vi "Parse Variable Value Pairs.vi"(10 "Value":string[](array[string])=["{a:757.273473m;b:445.885196m}", "306", "18", "106", "206", "454.112"], 11 "Name":string[](array[string])=["cluster", "intfromini", "response", "response1", "response2", "cluster.a"]) -> (2 "Value":string[](array[string])=["cluster", "cluster.a", "cluster.b", "intfromini", "response", "response1", "response2", "cluster.a"], 3 "Name2":string[](array[string])=["cluster", "cluster.a", "cluster.b", "intfromini", "response", "response1", "response2", "cluster.a"])   [LabVIEW 2020]
uses:
  <userlib>/_NEVSTOP/Communicable State Machine(CSM)/Communicable State Machine.lvlib
  <userlib>/_NEVSTOP/Communicable State Machine(CSM)/_Shared/CSM Shared.lvlib
panel:
  out "Indexs 2":dbl[](array[numeric])=[5.0, 0.0, 2.0, 3.0, 4.0, 5.0, 1.0] format="%.2f"
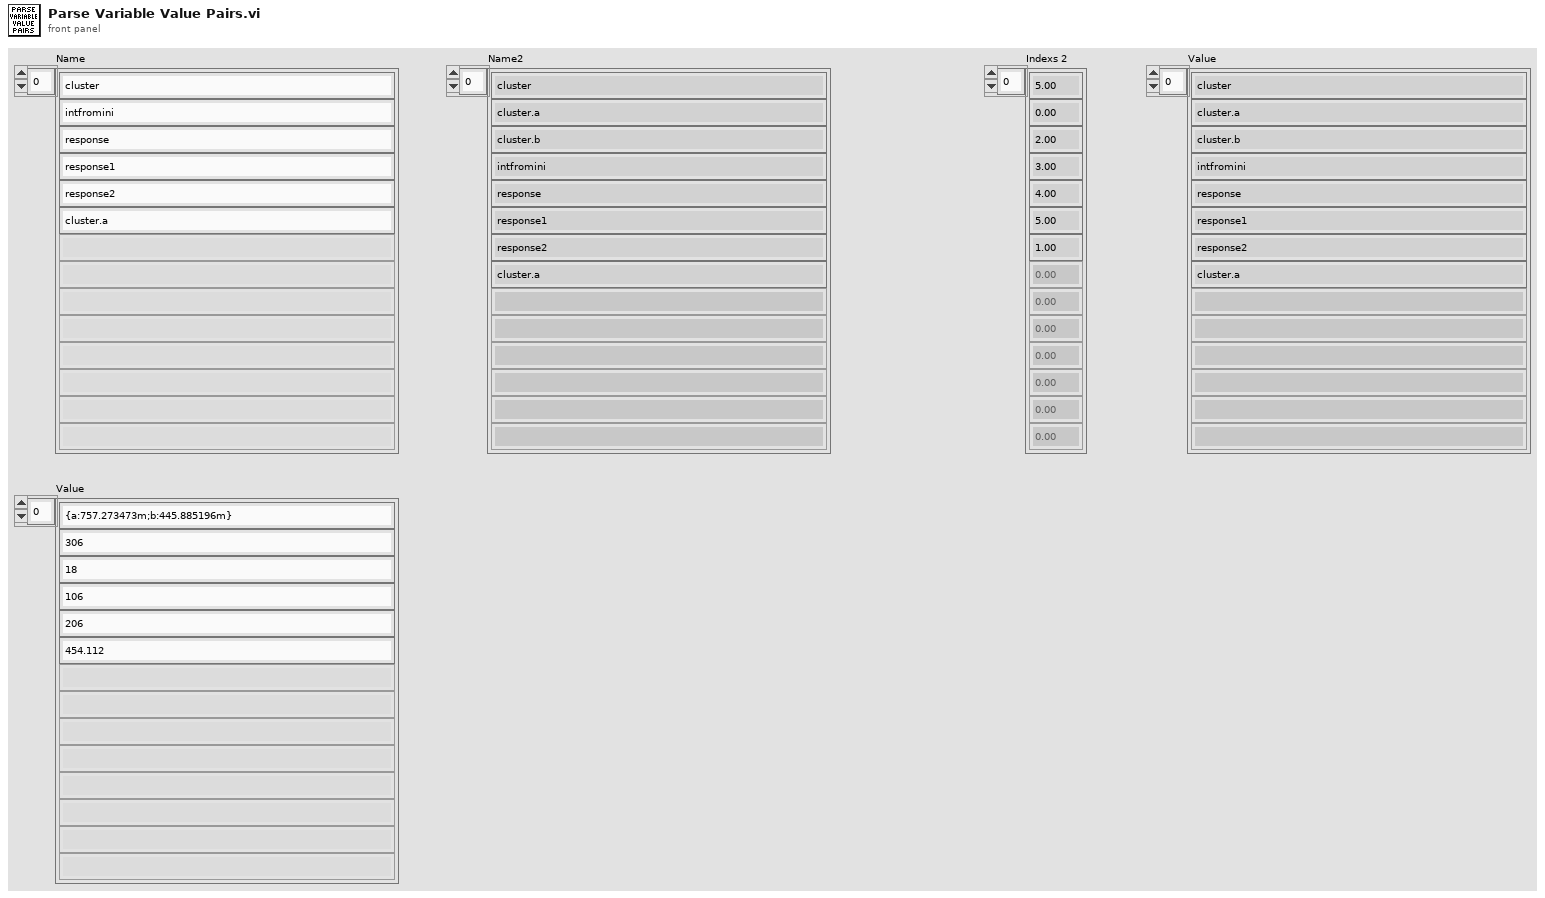
[diagram p1: front panel]
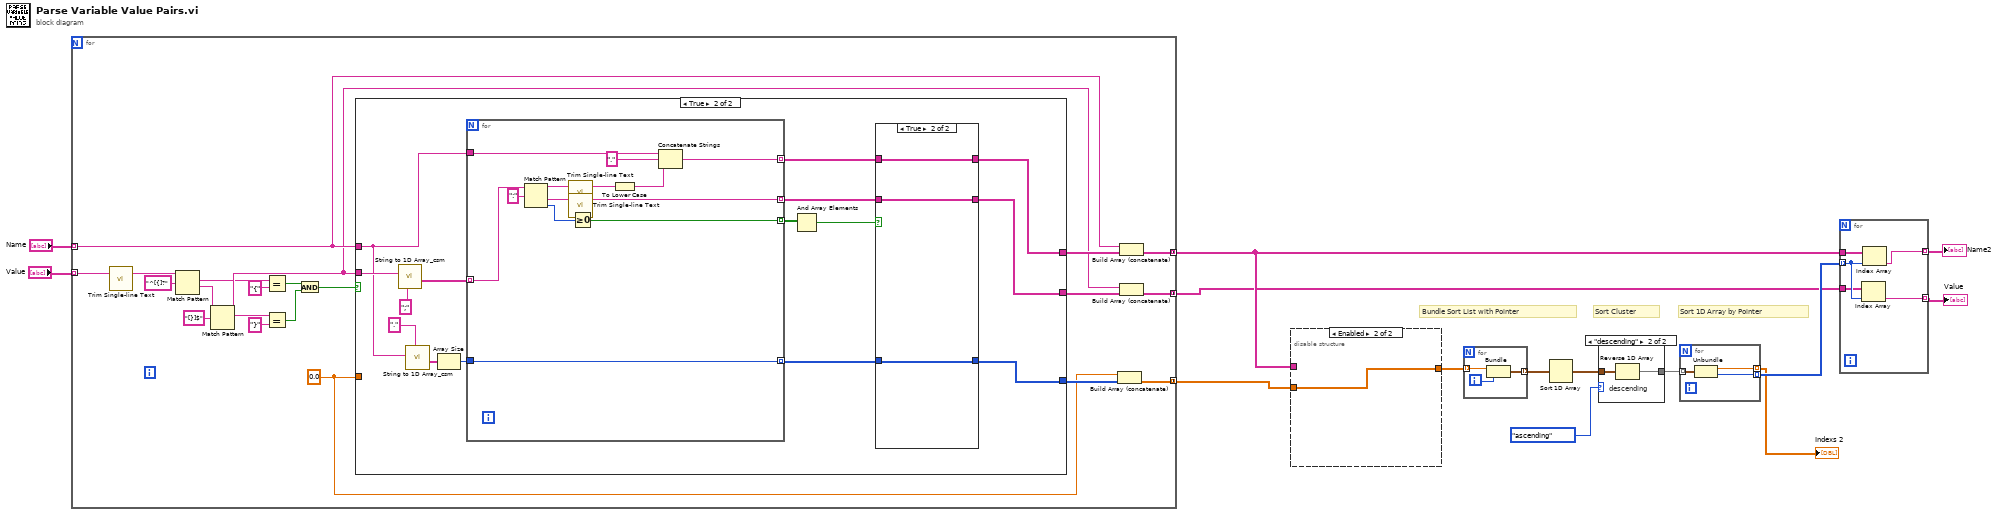
[diagram p0: block diagram]
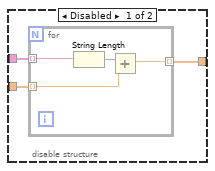
[diagram p2: hidden frame]
diagram:
  # "Sort 1D Array by Pointer"
  # "Sort Cluster"
  # "Bundle Sort List with Pointer"
  n1 = for {
    tunnel: "Value" -> [w35] mode=indexing
    tunnel: "Name" -> [w30] mode=indexing
    tunnel: [w32] -> w5 mode=concatenating
    tunnel: [w31] -> w2 mode=concatenating
    tunnel: [w23] -> w6 mode=concatenating
    w15 = 0.0 ("element")
    n2 = call <userlib>:"Trim Single-line Text.vi"("single-line text"=w35) -> ("trimed text"=w26:string)  [unwired: 2 in]
    n3 = Match Pattern(string=w26, regular expression="^[{]?") -> (match substring=w22:string, after substring=w27:string)  [unwired: 1 in, 2 out]
    n4 = Match Pattern(string=w27, regular expression="[}]$") -> (before substring=w25:string, match substring=w19:string)  [unwired: 1 in, 2 out]
    n5 = Equal?(x=w22, y="{" ("regular expression")) -> (x = y?=w18:bool)
    n6 = Equal?(x=w19, y="}" ("regular expression")) -> (x = y?=w17:bool)
    n7 = And(x=w18, y=w17) -> (x .and. y?=w16:bool)
    n8 = case shown="True" w16 {
      tunnel: [_ w39] -> w34
      tunnel: [_ w41] -> w33
      tunnel: w30 -> [_ w46]
      tunnel: w25 -> [_ w49]
      tunnel: [_ w37] -> w24
      tunnel: w15 -> [_ _]
      frame False {
      }
      frame True {
        n9 = call <userlib>:"String to 1D Array_csm.vi"("delimiter (Tab)"=";", "string"=w49) -> ("Array of Strings"=w48:string[])  [unwired: 9 in]
        n10 = call <userlib>:"String to 1D Array_csm.vi"("delimiter (Tab)"=".", "string"=w46) -> ("Array of Strings"=w45:string[])  [unwired: 9 in]
        n11 = Array Size(array=w45) -> (size(s)=w44:i32)
        n12 = for {
          tunnel: w48 -> [w61] mode=indexing
          tunnel: w46 -> [w60]
          tunnel: [w59] -> w43 mode=indexing
          tunnel: w44 -> [w58]
          tunnel: [w58] -> w36 mode=indexing
          tunnel: [w57] -> w40 mode=indexing
          tunnel: [w56] -> w38 mode=indexing
          n13 = Match Pattern(string=w61, regular expression=":") -> (before substring=w65:string, after substring=w63:string, offset past match=w64:i32)  [unwired: 1 in, 1 out]
          n14 = call <userlib>:"Trim Single-line Text.vi"("single-line text"=w65) -> ("trimed text"=w55:string)  [unwired: 2 in]
          n15 = call <userlib>:"Trim Single-line Text.vi"("single-line text"=w63) -> ("trimed text"=w57:string)  [unwired: 2 in]
          n16 = Greater Or Equal To 0?(x=w64) -> (x >= 0?=w59:bool)
          n17 = To Lower Case(string=w55) -> (all lower case string=w54:string)
          n18 = Concatenate Strings(w60, "." ("string"), w54) -> (w56:string)
        }
        n19 = And Array Elements(Boolean array=w43) -> (logical AND=w42:bool)
        n20 = case shown="True" w42 {
          tunnel: [_ w53] -> w41
          tunnel: w40 -> [_ w53]
          tunnel: [_ w52] -> w39
          tunnel: w38 -> [_ w52]
          tunnel: [_ w51] -> w37
          tunnel: w36 -> [_ w51]
          frame False {
          }
          frame True {
          }
        }
      }
    }
    n21 = Build Array (concatenate)(w15, w24) -> (w23:dbl[])
    n22 = Build Array (concatenate)(w30, w34) -> (w32:string[])
    n23 = Build Array (concatenate)(w25, w33) -> (w31:string[])
  }
  n24 = disable-structure shown="Enabled" {
    disable-tunnel: [w69 w74] -> w10
    disable-tunnel: w6 -> [w68 w74]
    disable-tunnel: w5 -> [w67 _]
    frame Disabled {
      n25 = for {
        tunnel: w67 -> [w73] mode=indexing
        tunnel: [w72] -> w69 mode=indexing
        tunnel: w68 -> [w70] mode=indexing
        n26 = String Length(string=w73) -> (length=w71:i32)
        n27 = Add(x=w71, y=w70) -> (x+y=w72:dbl)
      }
    }
    frame Enabled {
    }
  }
  n28 = for {
    tunnel: w10 -> [w77] mode=indexing
    tunnel: [w75] -> w13 mode=indexing
    i -> [w76]
    n29 = Bundle("element"=w77, w76) -> (w75:cluster{"element":dbl, i32})  [unwired: 1 in]
  }
  n30 = Sort 1D Array(array=w13) -> (sorted array=w12:cluster{"element":dbl, i32}[])
  n31 = case shown="\"descending\"" enum16{"ascending", "descending"}."ascending" ("Order") {
    tunnel: [w78 w79] -> w14
    tunnel: w12 -> [w78 w80]
    frame "ascending", Default {
    }
    frame "descending" {
      # "descending"
      n32 = Reverse 1D Array(array=w80) -> (reversed array=w79:cluster{"element":dbl, i32}[])
    }
  }
  n33 = for {
    tunnel: w14 -> [w83] mode=indexing
    tunnel: [w81] -> w3 mode=indexing
    tunnel: [w82] -> w11 mode=indexing
    n34 = Unbundle(w83) -> ("element"=w81:dbl, w82:i32)
  }
  "Indexs 2" <- w3
  n35 = for {
    tunnel: w5 -> [w88]
    tunnel: [w87] -> w4 mode=indexing
    tunnel: w11 -> [w86] mode=indexing
    tunnel: [w84] -> w1 mode=indexing
    tunnel: w2 -> [w85]
    n36 = Index Array(array=w85, index=w86) -> (element=w84:string)
    n37 = Index Array(array=w88, index=w86) -> (element=w87:string)
  }
  "Name2" <- w4
  "Value" <- w1
